vi "BRig_RT__Case_Exp__State_initTrial2__Laser_Power.vi"(0 "input_L_Power_max__x100":u16, 1 "input_LaserSwitch":bool, 5 "input_L_Power_min__x100":u16, 7 "input_L_Power_step__x100":u16) -> (6 "output_L_Power":dbl, 8 "output_L_Power_x100":u16)   [LabVIEW 2014]
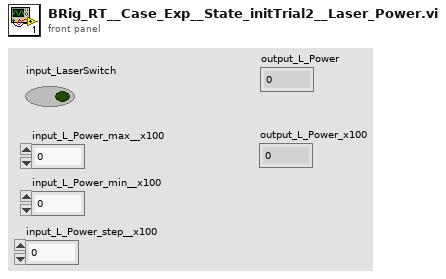
[diagram p1: front panel]
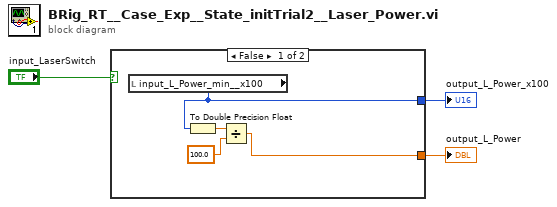
[diagram p0: block diagram]
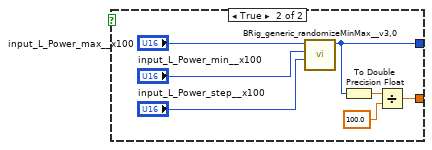
[diagram p2: hidden frame]
diagram:
  n1 = case shown="False" "input_LaserSwitch" {
    tunnel: [w5 w9] -> w2
    tunnel: [w4 w8] -> w1
    frame False {
      n2 = local read "input_L_Power_min__x100"() -> (w4:u16)
      n3 = To Double Precision Float(number=w4) -> (double precision float=w7:dbl)
      n4 = Divide(x=w7, y=100.0) -> (x/y=w5:dbl)
    }
    frame True {
      n5 = call "BRig_generic_randomizeMinMax__v3,0.vi"("Input_Increment"="input_L_Power_step__x100", "Input_Min"="input_L_Power_min__x100", "Input_Max"="input_L_Power_max__x100") -> ("Output"=w8:u16)  [unwired: 8 in]
      n6 = To Double Precision Float(number=w8) -> (double precision float=w11:dbl)
      n7 = Divide(x=w11, y=100.0) -> (x/y=w9:dbl)
    }
  }
  "output_L_Power" <- w2
  "output_L_Power_x100" <- w1
